vi "FlatToRichni_measurementlink_discovery_v1_EnumerateComputeNodesResponse.vi"(5 "OutputClusterType":T1, 11 "InputCluster":T3) -> (3 "OutputCluster":T1)   [LabVIEW 2024, in "ni.measurementlink.discovery.v1.api.lvlib"]
uses:
  ni.measurementlink.discovery.v1.api.lvlib
  ni_measurementlink_discovery_v1_EnumerateComputeNodesResponse_Flat.ctl
  ni_measurementlink_discovery_v1_ComputeNodeDescriptor_Flat.ctl
  ni_measurementlink_discovery_v1_EnumerateComputeNodesResponse.ctl
  ni_measurementlink_discovery_v1_ComputeNodeDescriptor.ctl
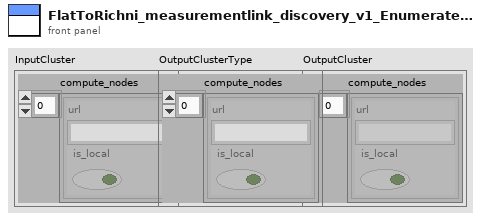
[diagram p1: front panel]
types:
  T1 = typedef "ni.measurementlink.discovery.v1.api.lvlib/ni_measurementlink_discovery_v1_EnumerateComputeNodesResponse.ctl" = cluster{"compute_nodes":T2[]}
  T2 = typedef "ni.measurementlink.discovery.v1.api.lvlib/ni_measurementlink_discovery_v1_ComputeNodeDescriptor.ctl" = cluster{"url":string, "is_local":bool}
  T3 = typedef "ni.measurementlink.discovery.v1.api.lvlib/ni_measurementlink_discovery_v1_EnumerateComputeNodesResponse_Flat.ctl" = cluster{"compute_nodes":T4[]}
  T4 = typedef "ni.measurementlink.discovery.v1.api.lvlib/ni_measurementlink_discovery_v1_ComputeNodeDescriptor_Flat.ctl" = cluster{"url":string, "is_local":bool}
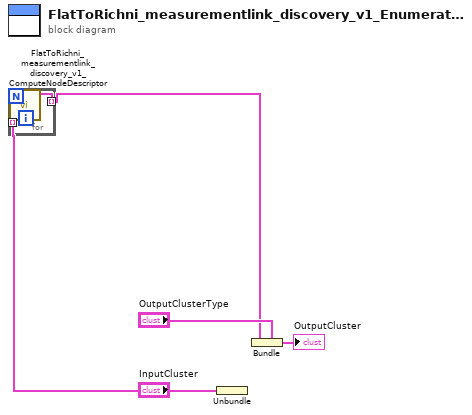
[diagram p0: block diagram]
diagram:
  n1 = Unbundle "Unbundle"("InputCluster") -> ("compute_nodes"=w2:T4[])
  n2 = for {
    tunnel: w2 -> [w7] mode=indexing
    tunnel: [w6] -> w1 mode=indexing
    n3 = call "FlatToRichni_measurementlink_discovery_v1_ComputeNodeDescriptor.vi"("InputCluster"=w7) -> ("OutputCluster"=w6:T2)  [unwired: 10 in]
  }
  n4 = Bundle "Bundle"(cluster="OutputClusterType", "compute_nodes"=w1) -> (→"OutputCluster":T1)
